vi "Field Generate Unique Record.vi"(8 "error in (no error)":errorcluster, 10 "Field Record (empty)":T2={"ixField"=0, "iSequenceOrder"=0, "sxFieldId"="", "sxSequenceId"="", "sDisplayName"="", "sValue"="", "sUnits"="", "nDataType"=enum."timestamp", "nNextItem"=enum."Reset", "fSystem"=FALSE, "fSystemValue"=FALSE, "fRequired"=FALSE, "fSetAtTest"=FALSE, "fTestField"=FALSE, "fDeleted"=FALSE, "fIndexed"=FALSE, "fFreeList"=FALSE}, 11 "Connection Refnum":T1) -> (0 "error out":errorcluster, 2 "Unique Field Record":T2={"ixField"=0, "iSequenceOrder"=0, "sxFieldId"="", "sxSequenceId"="", "sDisplayName"="", "sValue"="", "sUnits"="", "nDataType"=enum."timestamp", "nNextItem"=enum."Reset", "fSystem"=FALSE, "fSystemValue"=FALSE, "fRequired"=FALSE, "fSetAtTest"=FALSE, "fTestField"=FALSE, "fDeleted"=FALSE, "fIndexed"=FALSE, "fFreeList"=FALSE}, 3 "Connection Refnum":T1)   [LabVIEW 2011]
uses:
  Field Record.ctl
  Field DataTypes.ctl
  Field NextItem.ctl
  Summitek EXT/ODBC/SQL Controls/Connection Refnum.ctl
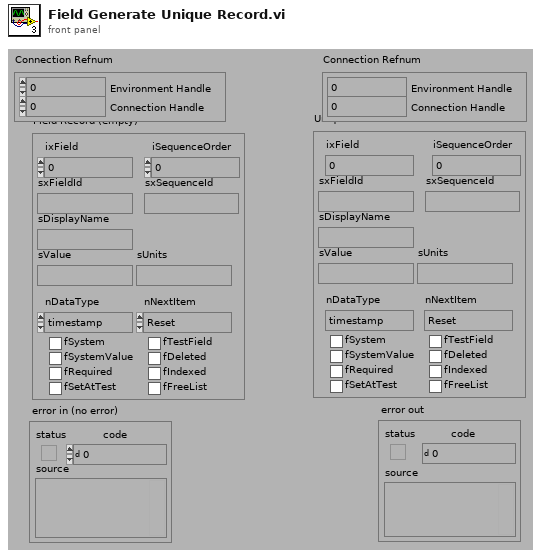
[diagram p1: front panel]
types:
  T1 = typedef "Connection Refnum.ctl" = cluster{"Environment Handle":i32, "Connection Handle":i32}
  T2 = typedef "Field Record.ctl" = cluster{"ixField":i32, "iSequenceOrder":i32, "sxFieldId":string, "sxSequenceId":string, "sDisplayName":string, "sValue":string, "sUnits":string, "nDataType":T3, "nNextItem":T4, "fSystem":bool, "fSystemValue":bool, "fRequired":bool, "fSetAtTest":bool, "fTestField":bool, "fDeleted":bool, "fIndexed":bool, "fFreeList":bool}
  T3 = typedef "Field DataTypes.ctl" = enum32{"text", "numeric", "list", "timestamp", "boolean"}
  T4 = typedef "Field NextItem.ctl" = enum32{"Reset", "Retain", "Auto-Increment"}
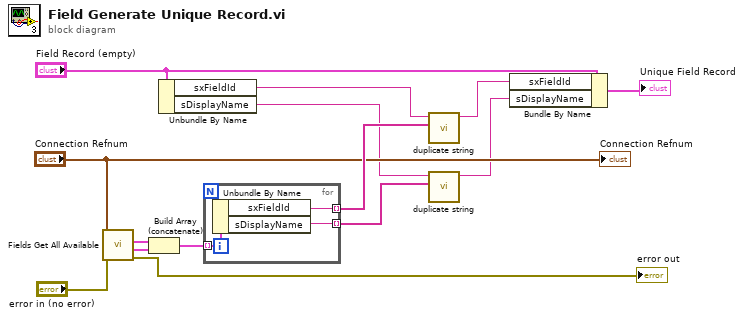
[diagram p0: block diagram]
diagram:
  n1 = call "Fields Get All Available.vi"("error in (no error)"="error in (no error)", "Connection Refnum"="Connection Refnum") -> ("error out"=→"error out":errorcluster, "Custom Fields"=w13:T2[], "System or ALL Combined Fields"=w14:T2[])  [unwired: 3 in, 4 out]
  n2 = Build Array (concatenate)(w14, w13) -> (w12:T2[])
  n3 = Unbundle By Name("Field Record (empty)") -> ("sxFieldId"=w4:string, "sDisplayName"=w2:string)
  n4 = for {
    tunnel: w12 -> [w17] mode=indexing
    tunnel: [w16] -> w11 mode=indexing
    tunnel: [w15] -> w10 mode=indexing
    n5 = Unbundle By Name(w17) -> ("sxFieldId"=w16:string, "sDisplayName"=w15:string)
  }
  n6 = call "duplicate string.vi"("Array of Strings"=w11, "String"=w4) -> ("Updated String"=w3:string)  [unwired: 9 out]
  n7 = call "duplicate string.vi"("Array of Strings"=w10, "String"=w2) -> ("Updated String"=w1:string)  [unwired: 9 out]
  n8 = Bundle By Name(cluster="Field Record (empty)", "sxFieldId"=w3, "sDisplayName"=w1) -> (→"Unique Field Record":T2)
  "Connection Refnum" <- "Connection Refnum"
